vi "readSingletime.vi"(8 "error in (no error)":errorcluster) -> (0 "error out":errorcluster, 3 "试验时间":dbl)   [LabVIEW 2014]
uses:
  <vilib>/addons/database/Connection.llb/DB Tools Open Connec (String).vi
  <vilib>/addons/database/Connection.llb/Conn Execute.vi
  <vilib>/addons/database/Recordset.llb/Rec Fetch Recordset Data (R).vi
  <vilib>/addons/database/Recordset.llb/Rec Destroy - Connection.vi
  <vilib>/addons/database/_DB Variant To Data/Database Variant To Data.xnode
  <vilib>/addons/database/NI_Database_API.lvlib
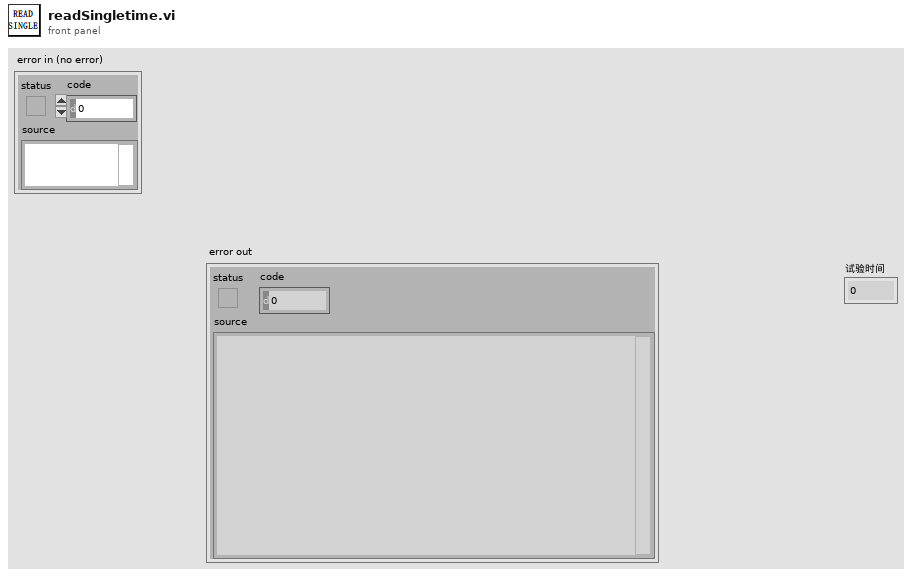
[diagram p1: front panel]
types:
  T1 = typedef "NI_Database_API.lvlib/Conn ObjectReference.ctl" = refnum<k1>
  T2 = typedef "NI_Database_API.lvlib/Rec ObjectReference.ctl" = refnum<k1>
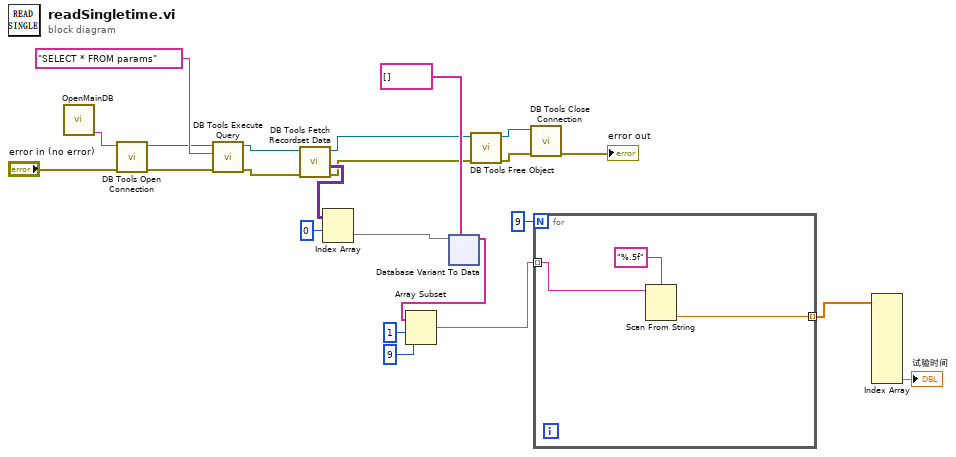
[diagram p0: block diagram]
diagram:
  n1 = call "OpenMainDB.vi"() -> ("头信息"=w2:string)  [unwired: 11 in]
  n2 = call-poly <vilib>:"DB Tools Open Connection.vi"("error in (no error)"="error in (no error)", "connection information"=w2) -> ("error out"=w6:errorcluster, "connection reference"=w5:T1)  [unwired: 6 in]
  n3 = call-poly <vilib>:"DB Tools Execute Query.vi"("error in (no error)"=w6, "SQL query"="SELECT * FROM params", "connection reference"=w5) -> ("error out"=w7:errorcluster, "recordset reference"=w4:T2)  [unwired: 5 in]
  n4 = call-poly <vilib>:"DB Tools Fetch Recordset Data.vi"("error in (no error)"=w7, "recordset reference"=w4) -> ("error out"=w10:errorcluster, "recordset data"=w14:variant[][], "recordset reference out"=w9:T2)  [unwired: 3 in]
  n5 = Index Array(array=w14, index (row)=0 ("索引 (行)")) -> (element=w16:variant[])  [unwired: 1 in]
  n6 = xnode "Database Variant To Data"("database variant"=w16, "type"=string[] []) -> ("data"=w20:string[])  [unwired: 1 in, 1 out]
  n7 = Array Subset(array=w20, index=1 ("索引"), length=9 ("长度")) -> (w23:string[])
  n8 = call-poly <vilib>:"DB Tools Free Object.vi"("error in (no error)"=w10, "recordset reference"=w9) -> ("error out"=w12:errorcluster, "connection reference"=w11:T1)  [unwired: 8 in]
  n9 = call <vilib>:"DB Tools Close Connection.vi"("error in (no error)"=w12, "connection reference"=w11) -> ("error out"=→"error out":errorcluster)  [unwired: 5 in]
  n10 = for {
    N: 9 -> [_]
    tunnel: w23 -> [w26] mode=indexing
    tunnel: [w24] -> w19 mode=indexing
    n11 = Scan From String(format string="%.5f" ("格式字符串"), input string=w26) -> (output 1=w24:dbl)  [unwired: 3 in, 3 out]
  }
  n12 = Index Array(array=w19) -> (element #9=→"试验时间":dbl)  [unwired: 9 in, 8 out]
